vi "Station_Wise_Enable_Disable_Para_Indi.vi"(6 "Communication Status Array":string[](array[string]), 8 "error in (no error)":errorcluster, 10 "?":T2={"Product List"=[], "SQL reference"=refnum, "Indicator refrence"=[], "Station Number"=[], "Shift Time stamp"=[timestamp(3597615000 s since 1904-01-01), timestamp(3597658199 s since 1904-01-01), timestamp(3597658200 s since 1904-01-01), timestamp(3597614999 s since 1904-01-01), timestamp(3597589800 s since 1904-01-01), timestamp(3597589800 s since 1904-01-01)], "Com Status Station"=[], "ALARAM INDICATOR REF"=[], "Reading"=[], "Read Parameteres"=[], "Station Name"=[], "Oven Read Parameteres"=[]} {"Shift Time stamp" format="%<%X>T"}, 11 "Parameter array":refnum<vi>[](array[refnum])) -> (0 "error out":errorcluster, 2 "Communication Status Array Out":string[](array[string]), 3 "Parameter array out":refnum<vi>[](array[refnum]))   [LabVIEW 2017]
doc: "This vi is used to diable the Parameter indicators in Station_Wise_VI AND this vi is used to name the indicator with station names"
uses:
  Controls/station_wise_loop_data.ctl
  <vilib>/addons/database/Connection.llb/Conn ObjectReference.ctl
  <vilib>/addons/database/NI_Database_API.lvlib
panel:
  out "Station Number":string[](array[string])
  in  "Para 1":T1
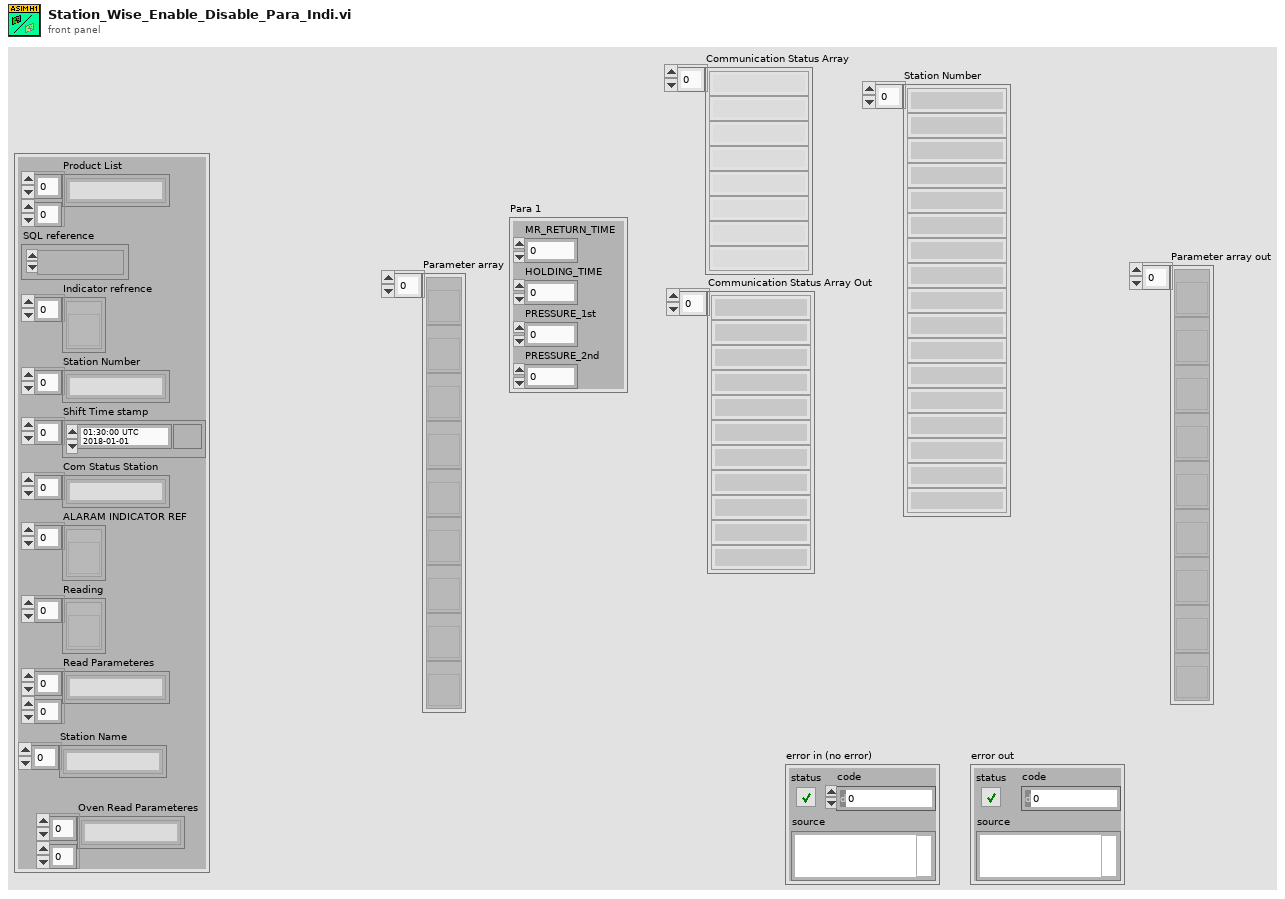
[diagram p1: front panel]
types:
  T1 = cluster{"MR_RETURN_TIME":dbl, "HOLDING_TIME":dbl, "PRESSURE_1st":dbl, "PRESSURE_2nd":dbl}
  T2 = typedef "station_wise_loop_data.ctl" = cluster{"Product List":string[][], "SQL reference":T3, "Indicator refrence":refnum<vi>[], "Station Number":string[], "Shift Time stamp":timestamp[], "Com Status Station":string[], "ALARAM INDICATOR REF":refnum<vi>[], "Reading":refnum<vi>[], "Read Parameteres":string[][], "Station Name":string[], "Oven Read Parameteres":string[][]}
  T3 = typedef "NI_Database_API.lvlib/Conn ObjectReference.ctl" = refnum<k1>
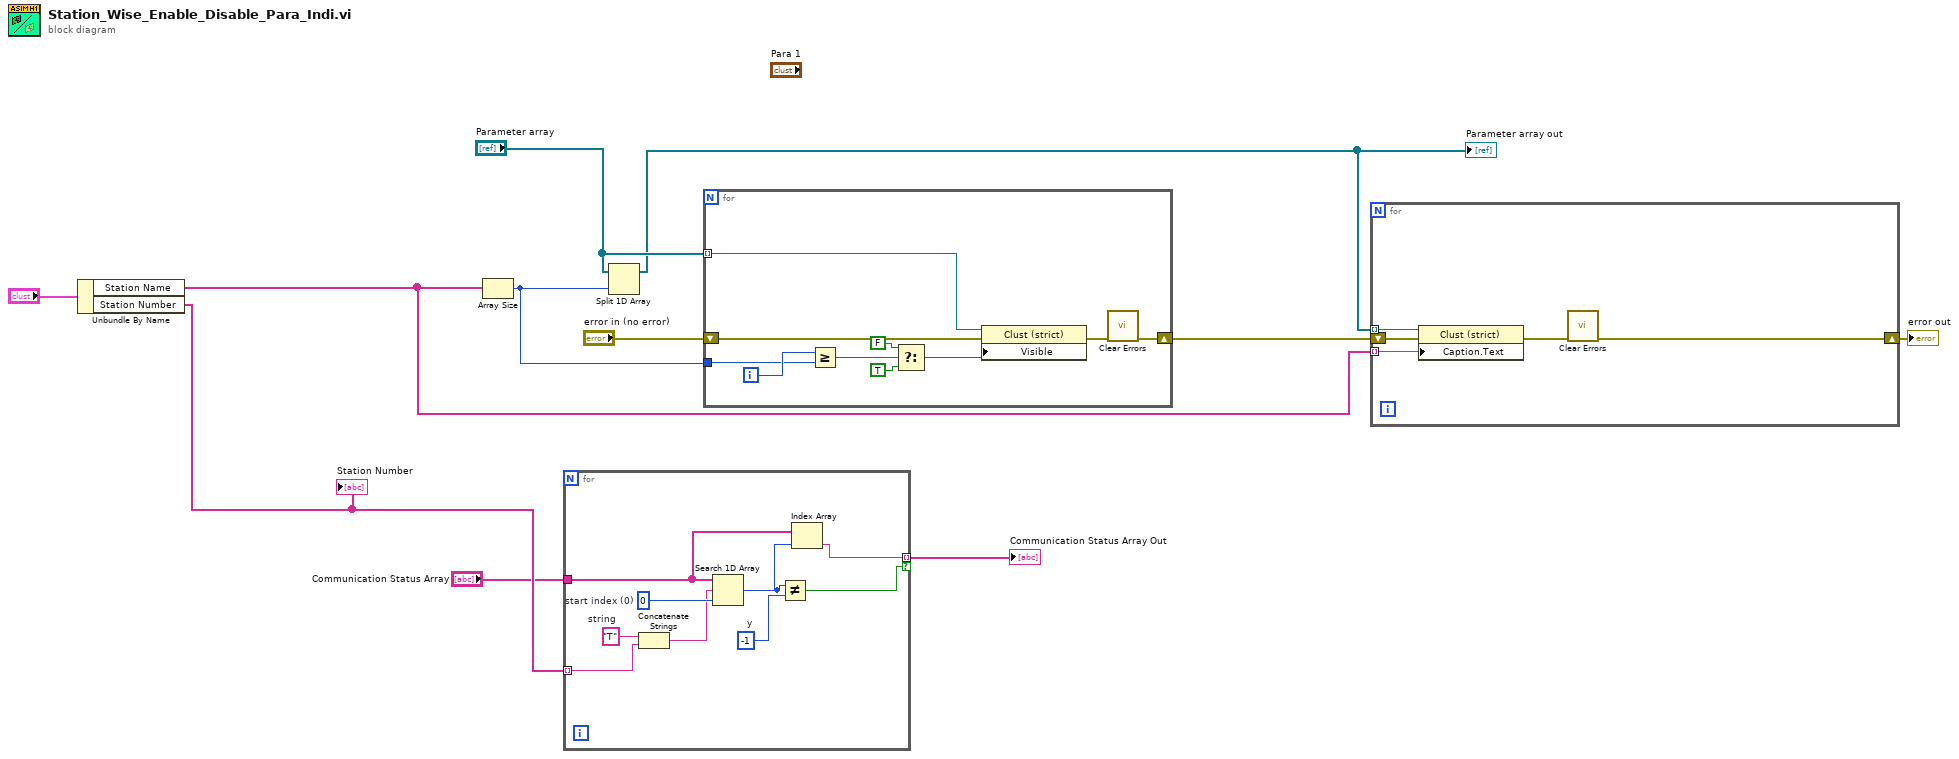
[diagram p0: block diagram]
diagram:
  n1 = Unbundle By Name("?") -> ("Station Name"=w4:string[], "Station Number"=w3:string[])
  "Station Number" <- w3
  n2 = Array Size(array=w4) -> (size(s)=w10:i32)
  n3 = for {
    tunnel: [w17] -> w1 mode=indexing if=w19
    tunnel: w3 -> [w13] mode=indexing
    tunnel: "Communication Status Array" -> [w14]
    w15 = 0  # start index (0)
    w16 = "T"  # string
    w20 = -1  # y
    n4 = Concatenate Strings(w16, w13) -> (w12:string)
    n5 = Search 1D Array(1D array=w14, element=w12, start index (0)=w15) -> (index of element=w18:i32)
    n6 = Not Equal?(x=w18, y=w20) -> (x != y?=w19:bool)
    n7 = Index Array(array=w14, index=w18) -> (element=w17:string)
  }
  "Communication Status Array Out" <- w1
  n8 = Split 1D Array(array="Parameter array", index=w10) -> (first subarray=w5:refnum<vi>[])  [unwired: 1 out]
  "Parameter array out" <- w5
  n9 = for {
    shift-right: [w21] -> w7
    shift-left: "error in (no error)" -> [w30]
    tunnel: "Parameter array" -> [w22] mode=indexing
    tunnel: w10 -> [w27]
    i -> [w28]
    n10 = Greater Or Equal?(x=w28, y=w27) -> (x >= y?=w26:bool)
    n11 = Select(t=FALSE, s=w26, f=TRUE) -> (s? t:f=w23:bool)
    n12 = property on="Property Node" class="Clust (strict)"(reference=w22, error in=w30, "Visible"=w23) -> (error out=w29:errorcluster)  [unwired: 1 out]
    n13 = call <vilib>:"Clear Errors.vi"("error in (no error)"=w29) -> ("error out"=w21:errorcluster)  [unwired: 5 in, 1 out]
  }
  n14 = for {
    shift-right: [w31] -> w6
    shift-left: w7 -> [w35]
    tunnel: w4 -> [w33] mode=indexing
    tunnel: w5 -> [w32] mode=indexing
    n15 = property on="Property Node" class="Clust (strict)"(reference=w32, error in=w35, "Caption.Text"=w33) -> (error out=w34:errorcluster)  [unwired: 1 out]
    n16 = call <vilib>:"Clear Errors.vi"("error in (no error)"=w34) -> ("error out"=w31:errorcluster)  [unwired: 5 in, 1 out]
  }
  "error out" <- w6
